vi "GoToDSM.vi"(8 "error in (no error)":errorcluster, 11 "Node Ptr":u64 format="%.0x") -> ()   [LabVIEW 2017, in "Shared Variables CD 2.0 Configuration.lvlib"]
uses:
  Shared Variables CD 2.0 Configuration.lvlib
  <vilib>/Utility/error.llb/Error Cluster From Error Code.vi
  <vilib>/ErrorRing/Error Ring.xnode
panel:
  in  "Tag":string
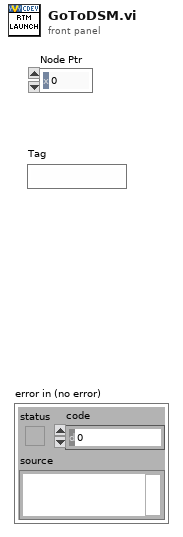
[diagram p1: front panel]
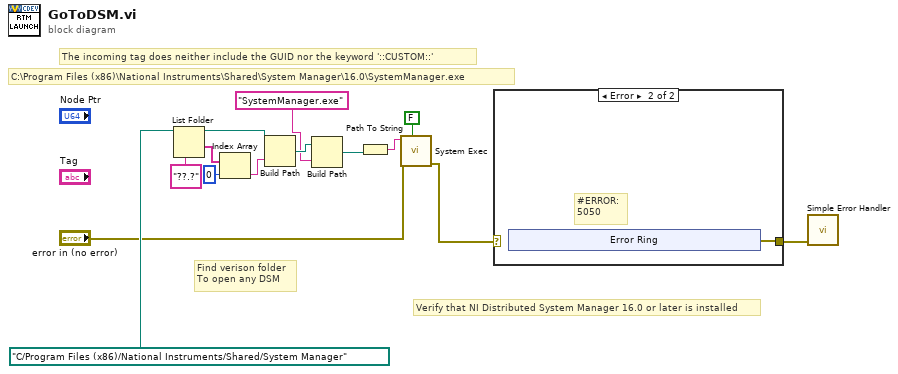
[diagram p0: block diagram]
diagram:
  # "Find verison folder\nTo open any DSM"
  # "Verify that NI Distributed System Manager 16.0 or later is installed"
  # "C:\\Program Files (x86)\\National Instruments\\Shared\\System Manager\\16.0\\SystemManager.exe"
  # "The incoming tag does neither include the GUID nor the keyword '::CUSTOM::'"
  n1 = List Folder(path=path "C:/Program Files (x86)/National Instruments/Shared/System Manager", pattern="??.?") -> (path out=w12:path, folder names=w7:string[])  [unwired: 2 in, 2 out]
  n2 = Index Array(array=w7, index=0) -> (element=w11:string)
  n3 = Build Path(base path=w12, name or relative path=w11) -> (appended path=w6:path)
  n4 = Build Path(base path=w6, name or relative path="SystemManager.exe" ("command line")) -> (appended path=w4:path)
  n5 = Path To String(path=w4) -> (string=w3:string)
  n6 = call <vilib>:"System Exec.vi"("wait until completion? (T)"=FALSE, "error in (no error)"="error in (no error)", "command line"=w3) -> ("error out"=w2:errorcluster)  [unwired: 5 in, 3 out]
  n7 = case shown="Error" w2 {
    selector: w2 -> [w15 _]
    tunnel: [w15 w16] -> w1
    frame No Error {
    }
    frame Error {
      # "#ERROR:\n5050"
      n8 = xnode "Error Ring"() -> ("error out"=w16:errorcluster)
    }
  }
  n9 = call <vilib>:"Simple Error Handler.vi"("error in (no error)"=w1) -> ()  [unwired: 4 in, 5 out]
